vi "Read Tag Data.vi"(8 "error in (no error)":errorcluster, 11 "Task D-O Channels":string[][](array[string])) -> (0 "error out":errorcluster, 3 "Array":bool[][](array[boolean]))   [LabVIEW 2021, in "DAQ.lvlib"]
uses:
  DAQ.lvlib
  Tag VIs/Tag FGV Operation Enum.ctl
  Shared Variables/Dynamic Shared Variables.lvlib
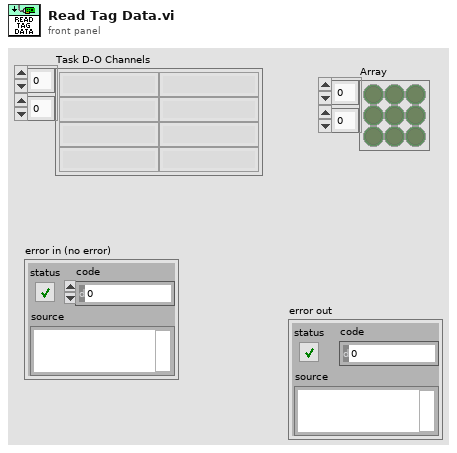
[diagram p1: front panel]
types:
  T1 = typedef "Tag FGV Operation Enum.ctl" = enum16{"Init", "Set Notification Queue", "Create Tag", "Commit", "Write Tag (Numeric)", "Write Tag (Boolean)", "Read All Tags", "Read One Tag", "Delete Tag Category", "Set Alarm Parameters (Numeric)", "Set Alarm Parameters (Boolean)", "Enable All Alarms", "Disable All Alarms", "Delete All Tags", "Read Alarms", "Ack Alarm", "Read Alarm Parameters (Numeric)", "Read Alarm Parameters (Boolean)"}
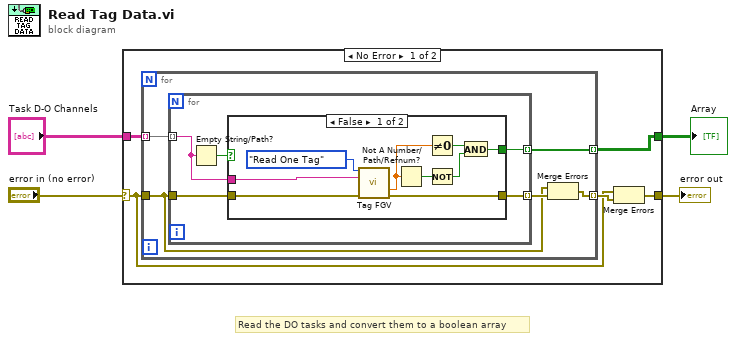
[diagram p0: block diagram]
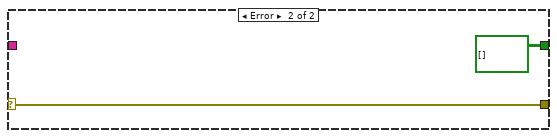
[diagram p3: hidden frame]
diagram:
  # "Read the DO tasks and convert them to a boolean array"
  n1 = case shown="No Error" "error in (no error)" {
    selector: "error in (no error)" -> [w6 w31]
    tunnel: [w5 w31] -> w4
    tunnel: "Task D-O Channels" -> [w9 _]
    tunnel: [w8 bool[][] []] -> w2
    frame No Error {
      n2 = for {
        tunnel: [w14] -> w7 mode=indexing
        tunnel: w9 -> [w11] mode=indexing
        tunnel: w6 -> [w10]
        tunnel: [w12] -> w8 mode=indexing
        n3 = for {
          tunnel: [w17] -> w12 mode=indexing
          tunnel: w11 -> [w15] mode=indexing
          tunnel: w10 -> [w19]
          tunnel: [w18] -> w13 mode=indexing
          n4 = Empty String/Path?(string/path=w15) -> (empty?=w16:bool)
          n5 = case shown="False" w16 {
            tunnel: w15 -> [w27 _]
            tunnel: w19 -> [w26 w29]
            tunnel: [w25 w29] -> w18
            tunnel: [w23 _] -> w17
            frame False {
              n6 = call "Tag FGV.vi"("Operation"=Tag_FGV_Operation_Enum."Read One Tag", "Tag Name"=w27, "error in (no error)"=w26) -> ("Tag Value"=w22:dbl, "error out"=w25:errorcluster)  [unwired: 5 in, 6 out]
              n7 = Not A Number/Path/Refnum?(number/path/refnum=w22) -> (NaN/Path/Refnum?=w21:bool)
              n8 = Not Equal To 0?(x=w22) -> (x != 0?=w24:bool)
              n9 = Not(x=w21) -> (.not. x?=w20:bool)
              n10 = And(x=w24, y=w20) -> (x .and. y?=w23:bool)
            }
            frame True {
            }
          }
        }
        n11 = Merge Errors(w10, w13) -> (w14:errorcluster)
      }
      n12 = Merge Errors(w6, w7) -> (w5:errorcluster)
    }
    frame Error {
    }
  }
  "error out" <- w4
  "Array" <- w2
